vi "Read Queue of Self Attributes.vi"(11 "Setup in":refnum<class "Setup.lvclass">) -> (2 "Queue of Self Attributes":refnum<queue>)   [LabVIEW 2025, in "jettl.lvlib" / "Setup.lvlib" / "Setup.lvclass"]
uses:
  Setup.lvclass
  Attributes/Attributes/Attributes.lvclass
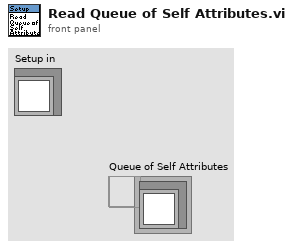
[diagram p1: front panel]
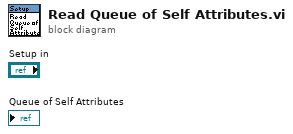
[diagram p0: block diagram]
diagram:
